vi "GenerateCollimationLightScanGrid.vi"(10 "扫描范围":dbl) -> (1 "纵向扫描位置":dbl[](array[numeric]), 2 "横向扫描位置":dbl[](array[numeric]))   [LabVIEW 2018]
panel:
  out "X":dbl
  out "Z":dbl
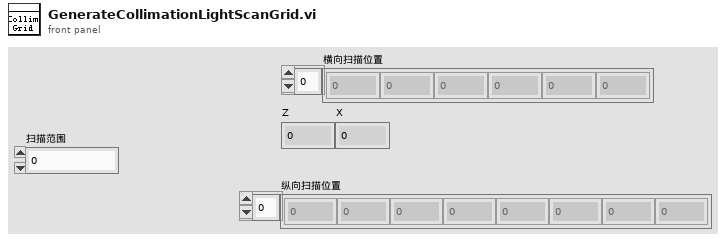
[diagram p1: front panel]
types:
  T1 = typedef "控制电机位置枚举器.ctl" = enum16{"远场扫描", "发散角扫描", "远场相机", "近场相机", "时间波形", "偏振", "能量", "功率", "光谱"}
  T2 = typedef "控制电机枚举器.ctl" = enum16{"Z", "Y", "X", "发散角", "俯仰", "旋转"}
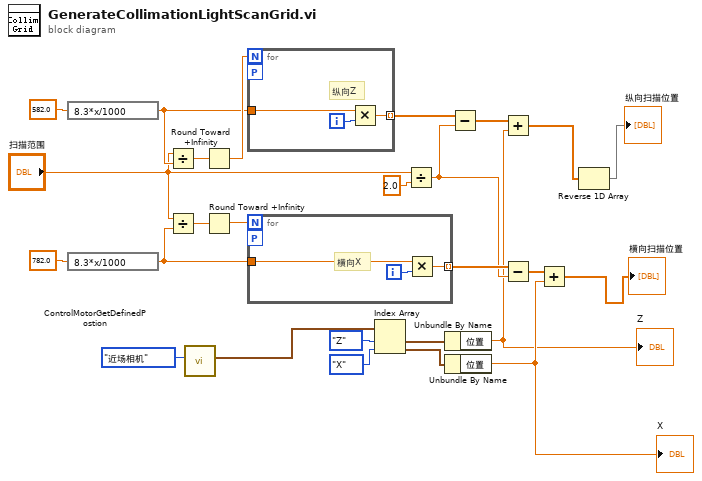
[diagram p0: block diagram]
diagram:
  n1 = expression code="8.3*x/1000"(582.0) -> (w19:dbl)
  n2 = expression code="8.3*x/1000"(782.0) -> (w22:dbl)
  n3 = Divide(x="扫描范围", y=w19) -> (x/y=w21:dbl)
  n4 = Divide(x="扫描范围", y=w22) -> (x/y=w24:dbl)
  n5 = call "ControlMotorGetDefinedPostion.vi"("位置"=控制电机位置枚举器."近场相机") -> ("PosOut"=w1:cluster{"控制电机":T2, "位置":dbl}[])  [unwired: 10 in]
  n6 = Round Toward +Infinity(x=w21) -> (ceil(x): smallest int >= x=w20:dbl)
  n7 = Round Toward +Infinity(x=w24) -> (ceil(x): smallest int >= x=w23:dbl)
  n8 = for {
    N: w20 -> [_]
    tunnel: w19 -> [w28]
    tunnel: [w27] -> w15 mode=indexing
    workers-P: _ -> [_]
    i -> [w29]
    # "纵向Z"
    n9 = Multiply(x=w28, y=w29) -> (x*y=w27:dbl)
  }
  n10 = for {
    N: w23 -> [_]
    tunnel: w22 -> [w32]
    tunnel: [w31] -> w16 mode=indexing
    workers-P: _ -> [_]
    i -> [w30]
    # "横向X"
    n11 = Multiply(x=w32, y=w30) -> (x*y=w31:dbl)
  }
  n12 = Index Array(array=w1, index #1=控制电机枚举器."Z" ("控制电机"), index #2=控制电机枚举器."X" ("控制电机")) -> (element #1=w11:cluster{"控制电机":T2, "位置":dbl}, element #2=w10:cluster{"控制电机":T2, "位置":dbl})
  n13 = Divide(x="扫描范围", y=2.0) -> (x/y=w14:dbl)
  n14 = Unbundle By Name(w11) -> ("位置"=w6:dbl)
  "Z" <- w6
  n15 = Unbundle By Name(w10) -> ("位置"=w8:dbl)
  "X" <- w8
  n16 = Subtract(x=w15, y=w14) -> (x-y=w7:dbl[])
  n17 = Add(x=w7, y=w6) -> (x+y=w5:dbl[])
  n18 = Subtract(x=w16, y=w14) -> (x-y=w9:dbl[])
  n19 = Add(x=w9, y=w8) -> (x+y=→"横向扫描位置":dbl[])
  n20 = Reverse 1D Array(array=w5) -> (reversed array=→"纵向扫描位置":dbl[])
